vi "MidbrainArbiter.vi"(0 "ForebrainInput":dbl[](array[numeric]), 5 "P-WallFollow":dbl[](array[numeric]), 7 "PushHome":dbl[](array[numeric]), 9 "SeekIR":dbl[](array[numeric]), 11 "ObsAvoid":dbl[](array[numeric]), 12 "AvoidWall":dbl[](array[numeric])) -> (4 "ActCommand":cluster{"Rudder":i32, "Propeller":i32})   [LabVIEW 2011]
doc: "This VI arbitrates the one command input form the Forebrain, and a set of inputs from the Limbic and Cerrebellum THINK processes and conducts a voting poll arbitor with input from each to determine the one output command.\n\nInputs: 90 cell arrays of weighted direction commands \n\nOutput: Cluster of desried velocity and direction"
panel:
  out "BrainWave Waveform Graph":dbl[][](graph)
  # "This subVI takes the three\nACT commands; one from the forebrain \nand three from the Midbrain and\naverages them"
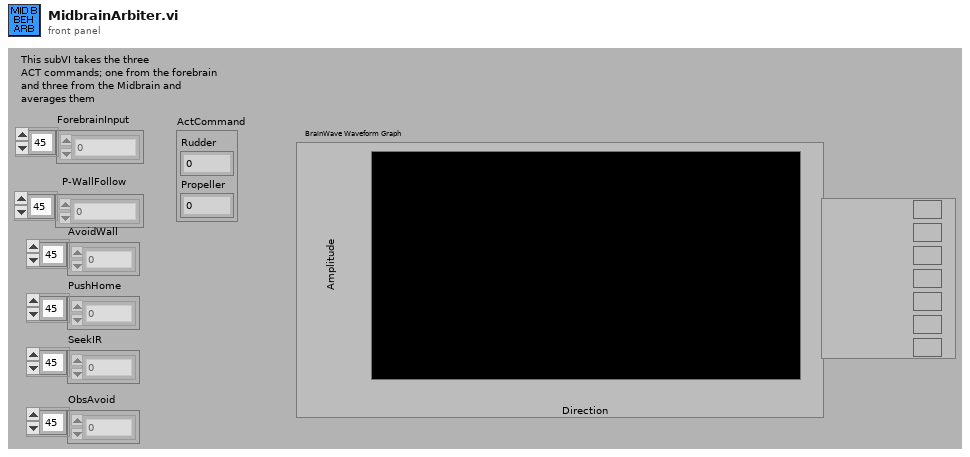
[diagram p1: front panel]
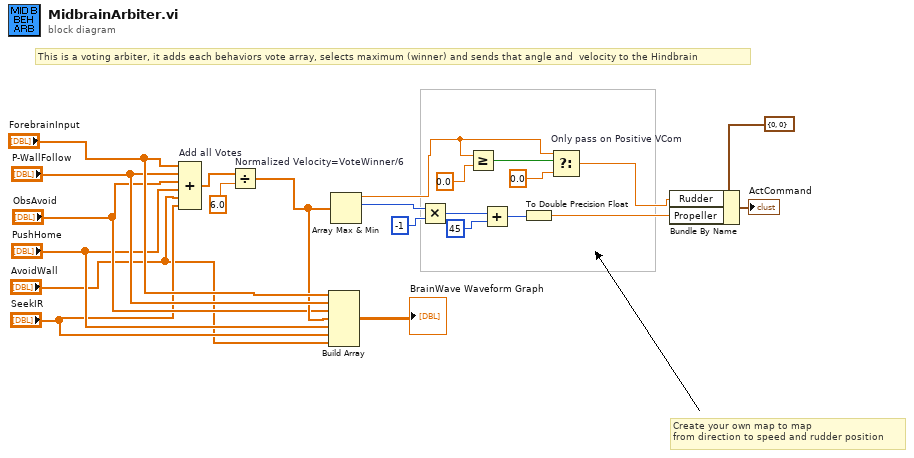
[diagram p0: block diagram]
diagram:
  # "Create your own map to map\nfrom direction to speed and rudder position"
  # "This is a voting arbiter, it adds each behaviors vote array, selects maximum (winner) and sends that angle and  velocity to the Hindbrain"
  n1 = Compound Arithmetic op=ADD "Add all Votes"("ForebrainInput", "P-WallFollow", "ObsAvoid", "PushHome", "AvoidWall", "SeekIR") -> (w13:dbl[])
  n2 = Divide "Normalized Velocity=VoteWinner/6"(x=w13, y=6.0) -> (x/y=w6:dbl[])
  n3 = Build Array "Build Array"("ForebrainInput", "P-WallFollow", "ObsAvoid", w6, "PushHome", "SeekIR", "AvoidWall") -> (→"BrainWave Waveform Graph":dbl[][])
  n4 = Array Max & Min(array=w6) -> (max value=w9:dbl, max index (indices)=w22:i32)  [unwired: 2 out]
  n5 = Multiply(x=w22, y=-1) -> (x*y=w20:i32)
  n6 = Greater Or Equal?(x=w9, y=0.0) -> (x >= y?=w10:bool)
  n7 = Add(x=w20, y=45) -> (x+y=w18:i32)
  n8 = To Double Precision Float(number=w18) -> (double precision float=w17:dbl)
  n9 = Select "Only pass on Positive VCom"(t=w9, s=w10, f=0.0) -> (s? t:f=w7:dbl)
  n10 = Bundle By Name(cluster=cluster{"Rudder":i32, "Propeller":i32} {"Rudder"=0, "Propeller"=0} ("Act Command"), "Rudder"=w7, "Propeller"=w17) -> (→"ActCommand":cluster{"Rudder":i32, "Propeller":i32})
